vi "Read Field.vi"(7 "field":string, 8 "error in (no error)":errorcluster, 11 "Base Interface in":refnum<class "Base Interface.lvclass">) -> (0 "error out":errorcluster, 2 "value":variant, 3 "Base Interface out":refnum<class "Base Interface.lvclass">)   [LabVIEW 2020, in "PV Access.lvlib" / "PV Data.lvlib" / "Base Interface.lvclass"]
doc: "Leave <B>field</B> blank to read the whole value."
uses:
  Base Interface.lvclass
  PV Data.lvlib
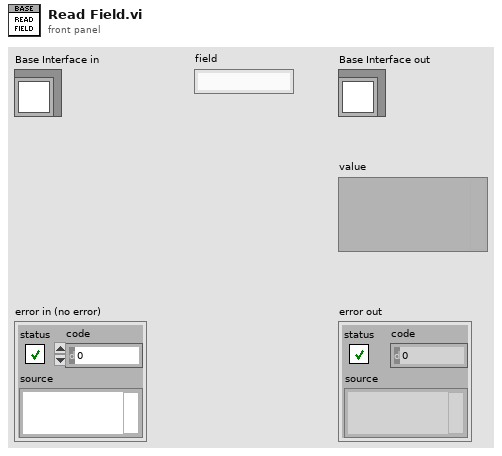
[diagram p1: front panel]
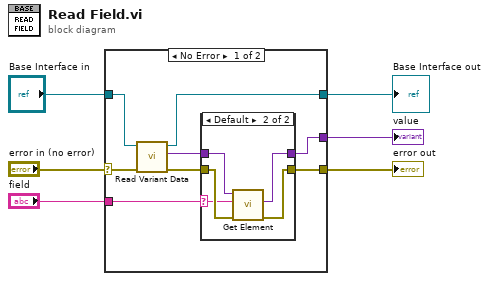
[diagram p0: block diagram]
diagram:
  n1 = case shown="No Error" "error in (no error)" {
    selector: "error in (no error)" -> [w13 w23]
    tunnel: [w10 w23] -> w3
    tunnel: [w12 w22] -> w5
    tunnel: "Base Interface in" -> [w14 w22]
    tunnel: "field" -> [w8 _]
    tunnel: [w7 _] -> w1
    frame No Error {
      n2 = call-dynamic "Read Variant Data.vi"("error in"=w13, "Base Interface in"=w14) -> ("error out"=w11:errorcluster, "data"=w9:variant, "Base Interface out"=w12:refnum<class "Base Interface.lvclass">)  [unwired: 7 in]
      n3 = case shown="Default" w8 {
        selector: w8 -> [_ w18]
        tunnel: w11 -> [w16 w21]
        tunnel: [w16 w20] -> w10
        tunnel: w9 -> [w15 w19]
        tunnel: [w15 w17] -> w7
        frame "" {
        }
        frame Default {
          n4 = call "Get Element.vi"("error in"=w21, "element name"=w18, "cluster in"=w19) -> ("error out"=w20:errorcluster, "element"=w17:variant)  [unwired: 6 in, 1 out]
        }
      }
    }
    frame Error {
    }
  }
  "error out" <- w3
  "Base Interface out" <- w5
  "value" <- w1
